vi "Resistivity2.vi"() -> ()   [LabVIEW 2017]
uses:
  <instrlib>/Keithley 6517/Keithley 6517.lvlib
panel:
  out "Resistivity":dbl
  in  "Area":dbl
  in  "Length":dbl format="%#_8f"
  out "units":string
  out "time stamp and date":string
  out "reading":dbl
  out "channel":dbl
  in  "Timeout(10000 ms)":u32=10000
  in  "source amplitude (2.0000000E+2)":dbl=200.0 format="%.7e"
  in  "Measurement Function (0: Resistance)":i32(ring) items=["Resistance", "Voltage", "Current", "Charge"]
  in  "VISA resource name 2":refnum<visa-resource-name>
  out "resistance":dbl format="%#_6f"
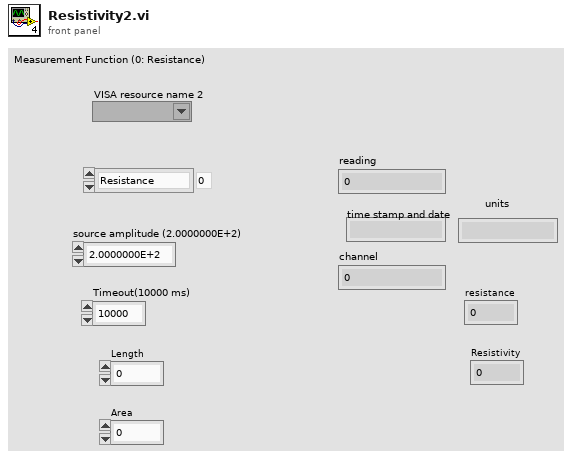
[diagram p1: front panel]
types:
  T1 = cluster{"Measurement":dbl, "Units":string, "Time Stamp and Date":string, "Reading #":dbl, "Channel #":dbl}
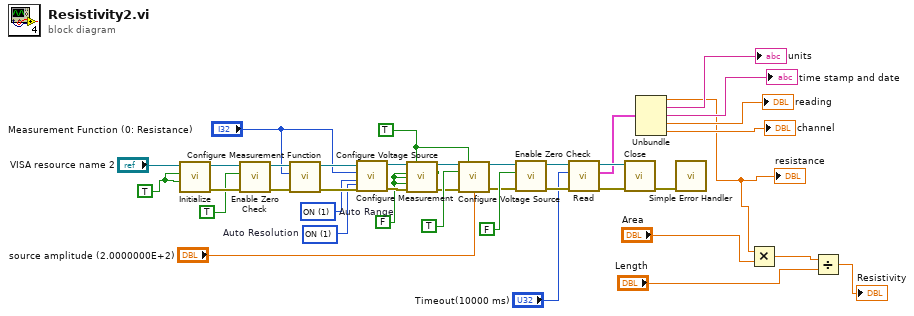
[diagram p0: block diagram]
diagram:
  w6 = TRUE
  w17 = FALSE
  w31 = 1 items=["OFF", "ON", "ONCE"]  # Auto Resolution
  w30 = 1 items=["OFF", "ON", "ONCE"]  # Auto Range
  w38 = TRUE
  n1 = call <instrlib>:"Initialize.vi"("Reset (True)"=w38, "ID Query (True)"=w38, "VISA resource name"="VISA resource name 2") -> ("error out"=w37:errorcluster, "VISA resource name out"=w36:refnum<visa-resource-name>)  [unwired: 7 in]
  n2 = call <instrlib>:"Enable Zero Check.vi"("error in (no error)"=w37, "Enable Zero Check (T: Enable)"=TRUE, "VISA resource name"=w36) -> ("error out"=w34:errorcluster, "VISA resource name out"=w35:refnum<visa-resource-name>)  [unwired: 7 in]
  n3 = call <instrlib>:"Configure Measurement Function.vi"("error in (no error)"=w34, "Measurement Function (0: Voltage)"="Measurement Function (0: Resistance)", "VISA resource name"=w35) -> ("error out"=w32:errorcluster, "VISA resource name out"=w33:refnum<visa-resource-name>)  [unwired: 7 in]
  n4 = call <instrlib>:"Configure Measurement.vi"("Auto Resolution (1: ON)"=w31, "error in (no error)"=w32, "Auto Range (1: ON)"=w30, "Measurement Function (0: Voltage)"="Measurement Function (0: Resistance)", "VISA resource name"=w33) -> ("error out"=w21:errorcluster, "VISA resource name out"=w22:refnum<visa-resource-name>)  [unwired: 5 in]
  n5 = call <instrlib>:"Configure Voltage Source.vi"("VISA resource name"=w22, "Enable LO Connection (F: Disable)"=w6, "Enable V-source (F: Disable)"=w17, "Enable Voltage Limit (F: Disable)"=w17, "Enable Resistance Current Limit (F: Disable)"=w17, "error in (no error)"=w21) -> ("VISA resource name out"=w20:refnum<visa-resource-name>, "error out"=w19:errorcluster)  [unwired: 8 in]
  n6 = call <instrlib>:"Configure Voltage Source.vi"("VISA resource name"=w20, "Enable LO Connection (F: Disable)"=w6, "Enable V-source (F: Disable)"=TRUE, "error in (no error)"=w19, "V-source Amplitude (0.000000E+0)"="source amplitude (2.0000000E+2)") -> ("VISA resource name out"=w25:refnum<visa-resource-name>, "error out"=w24:errorcluster)  [unwired: 9 in]
  n7 = call <instrlib>:"Enable Zero Check.vi"("error in (no error)"=w24, "Enable Zero Check (T: Enable)"=FALSE, "VISA resource name"=w25) -> ("error out"=w16:errorcluster, "VISA resource name out"=w15:refnum<visa-resource-name>)  [unwired: 7 in]
  n8 = call <instrlib>:"Read.vi"("error in (no error)"=w16, "Timeout(10000 ms)"="Timeout(10000 ms)", "VISA resource name"=w15) -> ("error out"=w14:errorcluster, "Measurement"=w7:T1, "VISA resource name out"=w13:refnum<visa-resource-name>)  [unwired: 6 in]
  n9 = call <instrlib>:"Close.vi"("error in (no error)"=w14, "VISA resource name"=w13) -> ("error out"=w27:errorcluster)  [unwired: 9 in]
  n10 = Unbundle(w7) -> ("Measurement"=w4:dbl, "Units"=→"units":string, "Time Stamp and Date"=→"time stamp and date":string, "Reading #"=→"reading":dbl, "Channel #"=→"channel":dbl)
  "resistance" <- w4
  n11 = call <vilib>:"Simple Error Handler.vi"("error in (no error)"=w27) -> ()  [unwired: 4 in, 5 out]
  n12 = Multiply(x=w4, y="Area") -> (x*y=w3:dbl)
  n13 = Divide(x=w3, y="Length") -> (x/y=→"Resistivity":dbl)
